vi "信息阅览.vi"() -> (11 "输出完毕":bool)   [LabVIEW 2023]
uses:
  e1efc265-fcc9-4f1c-a1a8-94133dad72b5.vi
  <vilib>/Array/Sort 2D Array - Pop Stack.vi
  <vilib>/Array/Sort 2D Array - Push Stack.vi
  <vilib>/Utility/file.llb/Read From Spreadsheet File (string).vi
panel:
  out "DCR_old":i32
  out "double_click_row":i32
  in  "返回":bool
  in  "排序":u16(ring) items=["默认", "学号", "寝室号"]
  in  "确认删除":bool
  in  "确认查询":bool
  in  "信息阅览":i32(listbox)
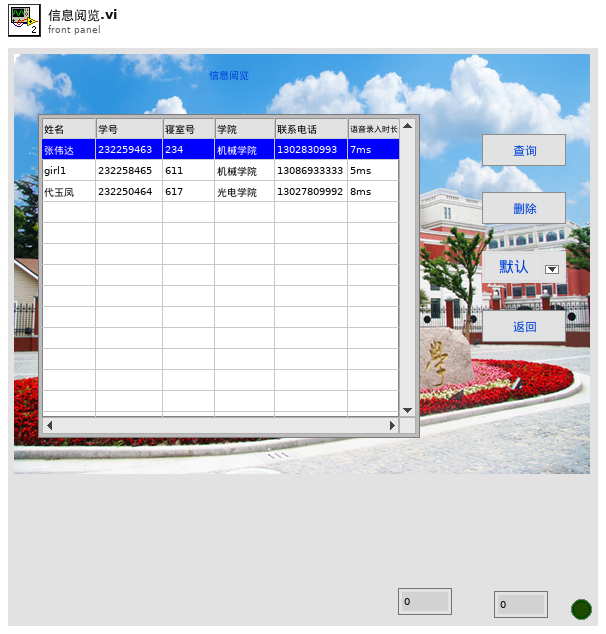
[diagram p1: front panel]
types:
  T1 = typedef "LVPoint32TypeDef.ctl" = cluster{"Horizontal":i32, "Vertical":i32}
  T2 = typedef "LVRowAndColumnTypeDef.ctl" = cluster{"Row":i32, "Column":i32}
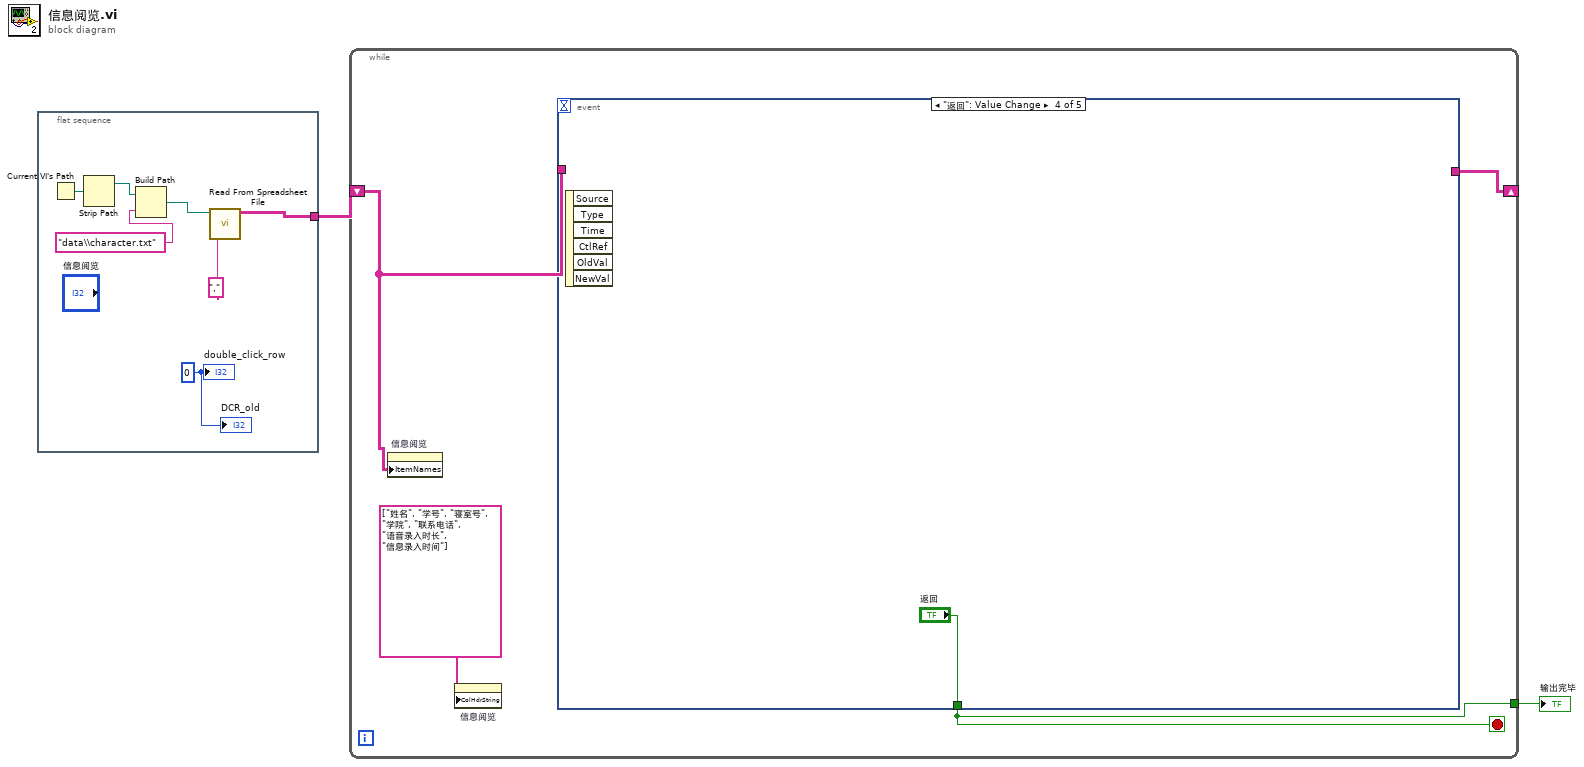
[diagram p0: block diagram]
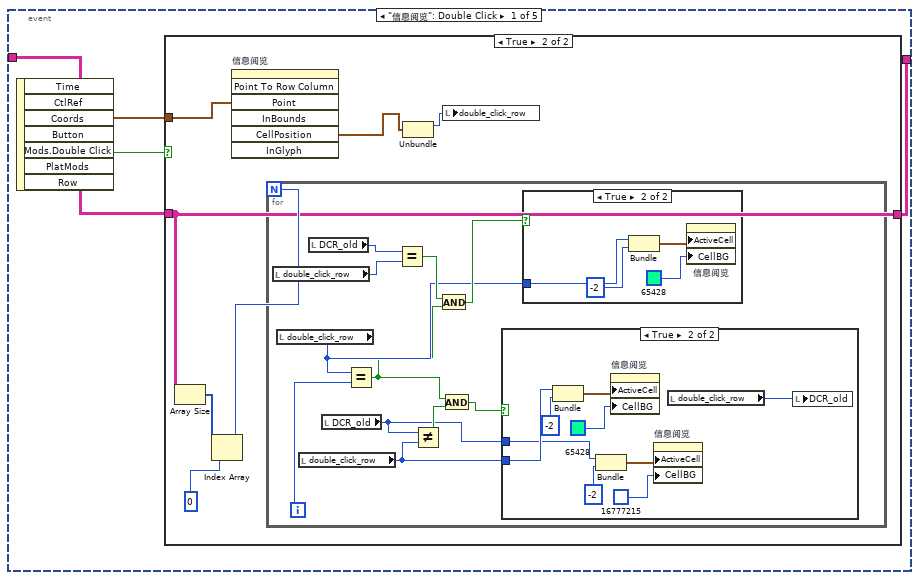
[diagram p2: hidden frame]
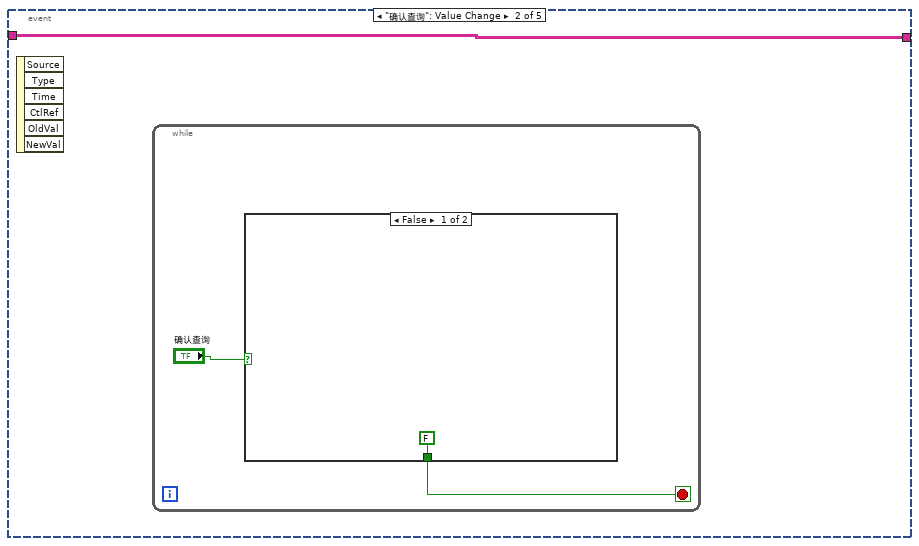
[diagram p6: hidden frame]
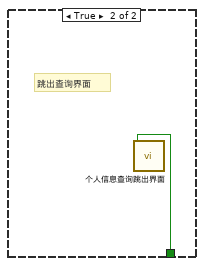
[diagram p7: hidden frame]
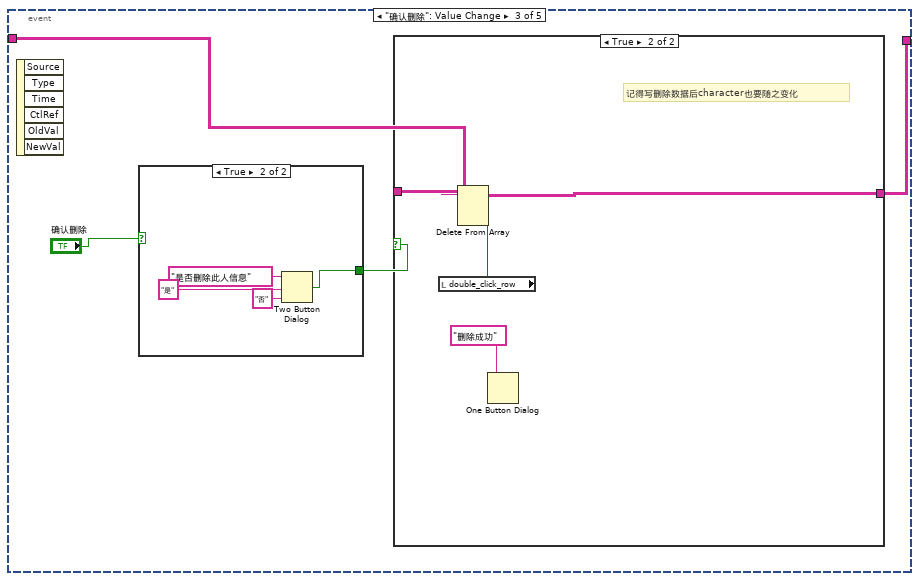
[diagram p8: hidden frame]
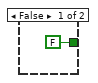
[diagram p10: hidden frame]
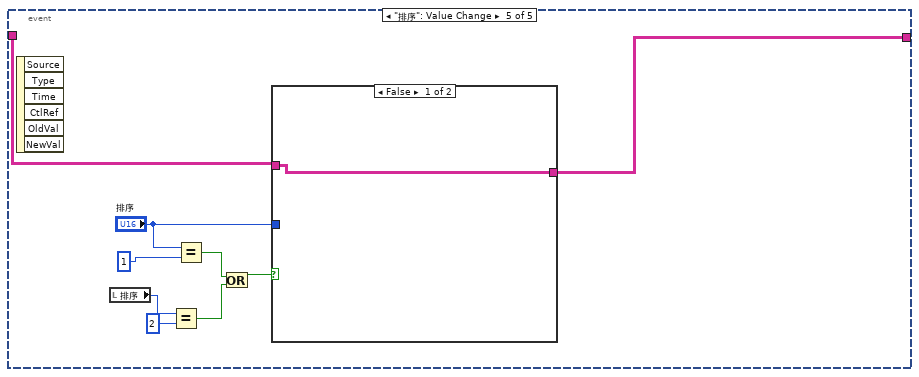
[diagram p11: hidden frame]
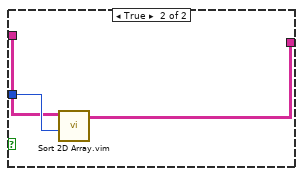
[diagram p12: hidden frame]
diagram:
  n1 = flat-sequence {
    tunnel: [w4] -> w2
    frame #0 {
      w3 = 0 ("double_click_row")
      n2 = Current VI's Path() -> (path=w9:path)
      n3 = Strip Path(path=w9) -> (stripped path=w8:path)  [unwired: 1 out]
      n4 = Build Path(base path=w8, name or relative path="data\\character.txt") -> (appended path=w5:path)
      n5 = call-poly <vilib>:"Read From Spreadsheet File.vi"("delimiter (\\t)"=",", "file path (dialog if empty)"=w5) -> ("all rows"=w4:string[][])  [unwired: 5 in, 4 out]
      "double_click_row" <- w3
      "DCR_old" <- w3
    }
  }
  n6 = while {
    shift-right: [w12] -> _
    shift-left: w2 -> [w13]
    tunnel: [w10] -> w1
    stop <- w10 stop-if-true
    n7 = property on="信息阅览" class="MCListbox (strict)"("ItemNames"=w13) -> ()  [unwired: 2 in, 2 out]
    n8 = property on="信息阅览" class="MCListbox (strict)"("ColHdrString"=string[] ["姓名", "学号", "寝室号", "学院", "联系电话", "语音录入时长", "信息录入时间"] ("Column Header Strings[]")) -> ()  [unwired: 2 in, 2 out]
    n9 = event shown="[3] \"返回\": Value Change" {
      selector: _ -> [_ _ _ _ _]
      dyn-events: _ -> [_ _ _ _ _]
      timeout: _ -> [_ _ _ _ _]
      tunnel: w13 -> [w15 w50 w56 _ w71]
      tunnel: [w14 w50 w55 _ w70] -> w12
      tunnel: [_ _ _ "返回" _] -> w10
      event "信息阅览": Double Click {
        n10 = event-data() -> ("Coords"=w16:T1, "Mods.Double Click"=w17:bool)  [unwired: 1 in, 5 out]
        n11 = case shown="True" w17 {
          tunnel: w16 -> [_ w25]
          tunnel: w15 -> [w18 w19]
          tunnel: [w18 w19] -> w14
          frame False {
          }
          frame True {
            n12 = Array Size(array=w19) -> (size(s)=w22:i32[])
            n13 = Index Array(array=w22, index=0) -> (element=w20:i32)
            n14 = invoke on="信息阅览" class="MCListbox (strict)" method="Point To Row Column"("Point"=w25) -> ("CellPosition"=w24:T2)  [unwired: 6 in, 6 out]
            n15 = for {
              N: w20 -> [_]
              i -> [w36]
              n16 = local read "double_click_row"() -> (w34:i32)
              n17 = local read "double_click_row"() -> (w31:i32)
              n18 = local read "double_click_row"() -> (w27:i32)
              n19 = local read "DCR_old"() -> (w35:i32)
              n20 = local read "DCR_old"() -> (w26:i32)
              n21 = Equal?(x=w31, y=w36) -> (x = y?=w30:bool)
              n22 = Equal?(x=w35, y=w34) -> (x = y?=w33:bool)
              n23 = Not Equal?(x=w26, y=w27) -> (x != y?=w29:bool)
              n24 = And(x=w33, y=w30) -> (x .and. y?=w32:bool)
              n25 = And(x=w30, y=w29) -> (x .and. y?=w28:bool)
              n26 = case shown="True" w28 {
                tunnel: w27 -> [_ w43]
                tunnel: w26 -> [_ w38]
                frame False {
                }
                frame True {
                  n27 = Bundle("double_click_row"=w43, -2) -> (w42:cluster{"double_click_row":i32, i32})  [unwired: 1 in]
                  n28 = Bundle("DCR_old"=w38, -2) -> (w39:cluster{"DCR_old":i32, i32})  [unwired: 1 in]
                  n29 = property on="信息阅览" class="MCListbox (strict)"("ActiveCell"=w42, "CellBG"=u32 65428) -> ()  [unwired: 2 in, 2 out]
                  n30 = property on="信息阅览" class="MCListbox (strict)"("ActiveCell"=w39, "CellBG"=u32 16777215) -> ()  [unwired: 2 in, 2 out]
                  n31 = local read "double_click_row"() -> (w37:i32)
                  n32 = local write "DCR_old"(w37) -> ()
                }
              }
              n33 = case shown="True" w32 {
                tunnel: w31 -> [_ w47]
                frame False {
                }
                frame True {
                  n34 = Bundle("double_click_row"=w47, -2) -> (w46:cluster{"double_click_row":i32, i32})  [unwired: 1 in]
                  n35 = property on="信息阅览" class="MCListbox (strict)"("ActiveCell"=w46, "CellBG"=u32 65428) -> ()  [unwired: 2 in, 2 out]
                }
              }
            }
            n36 = Unbundle(w24) -> ("Row"=w23:i32)  [unwired: 1 out]
            n37 = local write "double_click_row"(w23) -> ()
          }
        }
      }
      event "确认查询": Value Change {
        n38 = event-data() -> ()  [unwired: 1 in, 6 out]
        n39 = while {
          stop <- w51 stop-if-true
          n40 = case shown="False" "确认查询" {
            tunnel: [FALSE ("Boolean") w54] -> w51
            frame False {
            }
            frame True {
              # "跳出查询界面"
              n41 = call "个人信息查询跳出界面.vi"() -> ("Boolean"=w54:bool)  [unwired: 11 in]
            }
          }
        }
      }
      event "确认删除": Value Change {
        n42 = event-data() -> ()  [unwired: 1 in, 6 out]
        n43 = case shown="True" "确认删除" {
          tunnel: [FALSE ("T button?") w65] -> w57
          frame False {
          }
          frame True {
            n44 = Two Button Dialog(message="是否删除此人信息", 1:"否" ("F button name (\"Cancel\")"), 2:"是" ("T button name (\"OK\")")) -> (T button?=w65:bool)
          }
        }
        n45 = case shown="True" w57 {
          tunnel: w56 -> [w59 w63]
          tunnel: [w59 w62] -> w55
          frame False {
          }
          frame True {
            # "记得写删除数据后character也要随之变化"
            n46 = local read "double_click_row"() -> (w61:i32)
            n47 = Delete From Array(array=w63, index (row)=w61) -> (array with subset deleted=w62:string[][])  [unwired: 2 in, 1 out]
            n48 = One Button Dialog(message="删除成功") -> ()  [unwired: 1 in, 1 out]
          }
        }
      }
      event "返回": Value Change {
        n49 = event-data() -> ()  [unwired: 1 in, 6 out]
      }
      event "排序": Value Change {
        n50 = event-data() -> ()  [unwired: 1 in, 6 out]
        n51 = local read "排序"() -> (w77:u16)
        n52 = Equal?(x=w77, y=u16 2) -> (x = y?=w73:bool)
        n53 = Equal?(x="排序", y=1) -> (x = y?=w74:bool)
        n54 = Or(x=w74, y=w73) -> (x .or. y?=w75:bool)
        n55 = case shown="False" w75 {
          tunnel: "排序" -> [_ w82]
          tunnel: w71 -> [w79 w81]
          tunnel: [w79 w80] -> w70
          frame False {
          }
          frame True {
            n56 = call "Sort 2D Array.vim"("index"=w82, "2D array"=w81) -> ("sorted 2D array"=w80:string[][])  [unwired: 8 in, 1 out]
          }
        }
      }
    }
  }
  "输出完毕" <- w1
